vi "FFT_DAS Acq Thermocouple Sample.vi"() -> ()   [LabVIEW 2010]
doc: "I. Description:\nThis example demonstrates how to make temperature measurement using a thermocouple.\n\nII. Instructions for Running:\n1. Specify the Physical Channel where you have connected the thermocouple.\n2. Enter the Minimum and Maximum temperature values you expect to measure in degrees C. A smaller range will allow a more accurate measurement.\n3. Specify the type of thermocouple you are using.\n4. Thermocouple measurements require cold-junction compensation (CJC) to correctly scale them. Specify the source of your cold-junction compensation.\n5. If your CJC source is \"Internal\", skip the rest of steps.\n6. If your CJC source is \"Constant Value\", specify the value (usually room temperature) in degrees C.\n7. If your CJC source is \"Channel\", specify the CJC Channel name. \n\nIII. Block Diagram Steps:\n1. Create a Thermocouple (TC) temperature measurement channel.\n2. Call the Read VI to read one point of data.\n3. Call the Clear Task VI to clear the Task \n4. Use the popup dialog box to display an error if any.\n\nIV. I/O Connections Overview:\nConnect your thermocouple to the terminals corresponding to the Physical Channel I/O Control value."
uses:
  <vilib>/Utility/error.llb/DialogType.ctl
  <vilib>/Platform/TimedLoop/XDataNode/XDataNode.xnode
  <vilib>/Platform/TimedLoop/XDataNode/timing_clust.ctl
  <vilib>/Platform/TimedLoop/XDataNode/nitl_modes.ctl
  <vilib>/Platform/TimedLoop/XDataNode/wakeup.ctl
  <vilib>/DAQmx/read.llb/DAQmx Read (Analog DBL 1Chan 1Samp).vi
  <vilib>/DAQmx/create/channels.llb/DAQmx Create Channel (AI-Temperature-Thermocouple).vi
  <vilib>/daqmx/miscellaneous.llb/DAQmx Fill In Error Info.vi
  <vilib>/Platform/TimedLoop/XDataNode/XDNodeRunTimeDep.lvlib
panel:
  out "mSec":u32
  out "Loops":i32
  in  "stop":bool
  out "Measurement":cluster{"data":dbl, u32}(graph)
  in  "CJC Source":i32(ring)=10116 items=["Built-In"=10200, "Constant Value"=10116, "Channel"=10113]
  in  "Physical Channel":tag="Dev2/ai0"
  in  "Minimum value (deg C)":dbl format="%0.2f"
  in  "Maximum value (deg C)":dbl=100.0 format="%0.2f"
  in  "CJC Channel":refnum<k21>
  in  "CJC Value":dbl=25.0 format="%0.2f"
  in  "Thermocouple Type":i32(ring)=10072 items=["J"=10072, "K"=10073, "N"=10077, "R"=10082, "S"=10085, "T"=10086, "B"=10047, "E"=10055]
  out "Temperature":dbl(slide) scale=0.0..100.0
  # "For instructions, select Help>>Show Context Help"
  # "Channel Parameters"
  # "Cold Junction Parameters"
  # "Thermocouple Parameters"
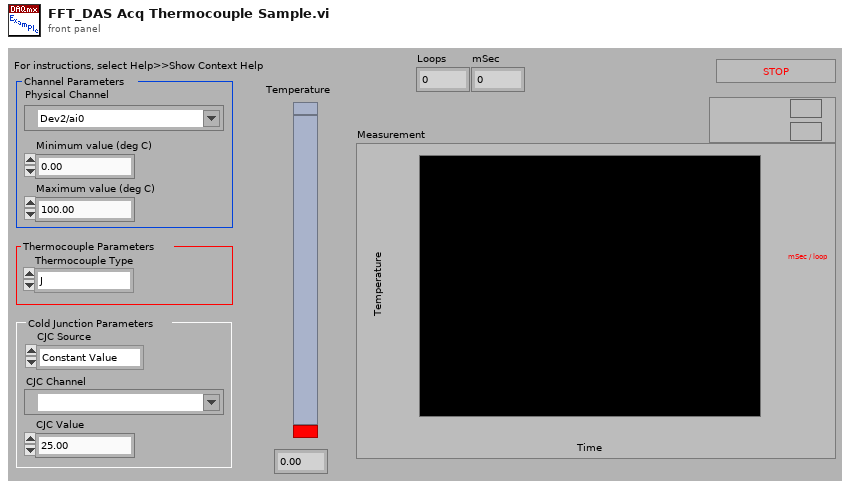
[diagram p1: front panel]
types:
  T1 = typedef "DialogType.ctl" = u16
  T2 = typedef "XDNodeRunTimeDep.lvlib/timing_clust.ctl" = cluster{"Expected End [f-1]":u64, "Actual End [f-1]":u64, "Finished Late? [f-1]":bool, "Expected End [i-1]":u64, "Actual End [i-1]":u64, "Finished Late? [i-1]":bool, "Expected Start [i]":u64, "Actual Start [i]":u64, "Expected Start [f]":u64, "Actual Start [f]":u64, "Source Name":string, "Structure Name":string, "Period":i64, "Deadline":i64, "Offset":i64, "Start":i64, "Priority":i32, "Timeout":i32, "Mode":T3, "Wakeup Reason":T4, "Error":errorcluster, "Source Type":string, "Secondary Source Type":string, "Global End Time":u64, "Global Start Time":u64, "Frame Duration":u64, "Iteration Duration":u64, "Assigned CPU":i32, "I/O Scan Engine Mode":u32}
  T3 = typedef "XDNodeRunTimeDep.lvlib/nitl_modes.ctl" = enum32{"No Change", "Process missed periods, maintain original phase", "Discard missed periods, maintain original phase", "Process missed periods, ignore original phase", "Discard missed periods, ignore original phase"}
  T4 = typedef "XDNodeRunTimeDep.lvlib/wakeup.ctl" = enum32{"Normal", "Aborted", "Asynchronous wakeup", "Timing source error", "Timed loop error", "Timeout"}
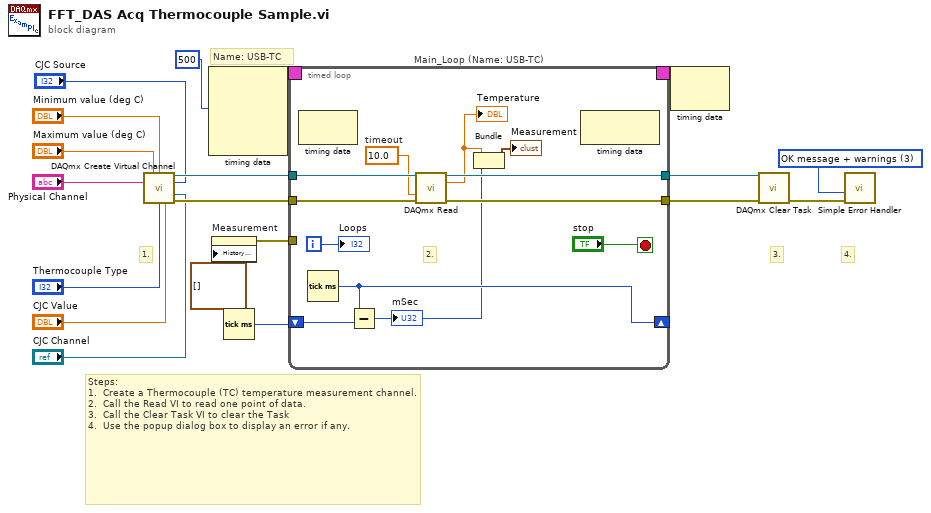
[diagram p0: block diagram]
diagram:
  w11 = T1 3 items=["no dialog", "OK message", "continue or stop message", "OK message + warnings", "continue/stop + warnings"] ("type of dialog (OK msg:1)")
  # "Name: USB-TC"
  # "3."
  # "4."
  # "1."
  # "Steps: \n1.  Create a Thermocouple (TC) temperature measurement channel.\n2.  Call the Read VI to read one point of data.\n3.  Call the Clear Task VI to clear the Task  \n4.  Use the popup dialog box to display an error if any."
  n1 = call-poly <vilib>:"DAQmx Create Virtual Channel.vi"("maximum value"="Maximum value (deg C)", "minimum value"="Minimum value (deg C)", "physical channels"="Physical Channel", "cjc source"="CJC Source", "cjc channel"="CJC Channel", "thermocouple type"="Thermocouple Type", "cjc value"="CJC Value") -> ("task out"=w19:refnum<k21>, "error out"=w18:errorcluster)  [unwired: 7 in]
  n2 = node-c288(i64 500 ("Period")) -> (w6:T2)  [unwired: 3 in]
  n3 = property on="Measurement" class="WFChart (strict)"("History Data"=cluster{"data":dbl, u32}[] []) -> (error out=w3:errorcluster)  [unwired: 2 in, 1 out]
  n4 = Tick Count (ms)() -> (millisecond timer value=w2:u32)
  n5 = timed-loop "Main_Loop (Name: USB-TC)" {
    timing: w6 -> [_]
    timing-out: [_] -> w5
    tunnel: w19 -> [w31]
    tunnel: w18 -> [w30]
    tunnel: [w28] -> w10
    tunnel: [w27] -> w9
    tunnel: w3 -> [_]
    shift-right: [w23] -> _
    shift-left: w2 -> [w24]
    i -> [w25]
    stop <- "stop" stop-if-true
    w29 = 10.0  # timeout
    # "2."
    n6 = node-c288() -> ()  [unwired: 1 in, 1 out]
    n7 = Tick Count (ms)() -> (millisecond timer value=w23:u32)
    n8 = Subtract(x=w23, y=w24) -> (x-y=w21:u32)
    "mSec" <- w21
    n9 = call-poly <vilib>:"DAQmx Read.vi"("task/channels in"=w31, "timeout"=w29, "error in"=w30) -> ("task out"=w28:refnum<k21>, "data"=w22:dbl, "error out"=w27:errorcluster)  [unwired: 10 in]
    "Temperature" <- w22
    n10 = Bundle("data"=w22, w21) -> (→"Measurement":cluster{"data":dbl, u32})  [unwired: 1 in]
    n11 = node-c288() -> ()  [unwired: 1 in, 1 out]
    "Loops" <- w25
  }
  n12 = node-c288(w5) -> ()  [unwired: 1 out]
  n13 = call <vilib>:"DAQmx Clear Task.vi"("task in"=w10, "error in"=w9) -> ("error out"=w8:errorcluster)  [unwired: 13 in]
  n14 = call <vilib>:"Simple Error Handler.vi"("type of dialog (OK msg:1)"=w11, "error in (no error)"=w8) -> ()  [unwired: 3 in, 5 out]
